vi "Write WaitStarted.vi"(10 "WaitStarted":bool, 11 "SMO.DynamicLauncher in":refnum<class "SMO.DynamicLauncher.lvclass">) -> (3 "SMO.DynamicLauncher out":refnum<class "SMO.DynamicLauncher.lvclass">)   [LabVIEW 2013, in "SMO.DynamicLauncher.lvclass"]
uses:
  SMO.DynamicLauncher.lvclass
  SMO.DynamicLauncher.lvclass/SMO.DynamicLauncher.ctl
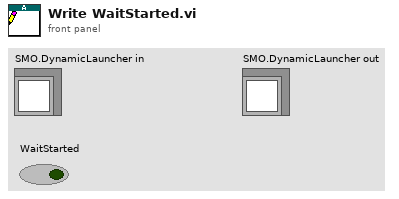
[diagram p1: front panel]
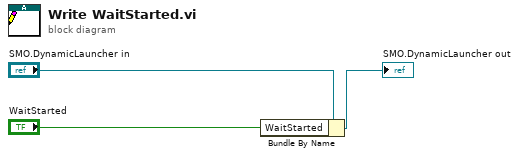
[diagram p0: block diagram]
diagram:
  n1 = Bundle By Name(cluster="SMO.DynamicLauncher in", "WaitStarted"="WaitStarted") -> (→"SMO.DynamicLauncher out":refnum<class "SMO.DynamicLauncher.lvclass">)
